vi "Emballage_BDD_option_Certificat.vi"(8 "Error in":errorcluster caption="Error in (no error)") -> (0 "Error out":errorcluster)   [LabVIEW 2020]
uses:
  Labview emballage/enum_ON_OFF_Lecteur.ctl
panel:
  in  "stop":bool
  in  "Bouton scanner":bool
  out "Code-barre":string
  # "Veuillez scanner le code-barre du produit!!"
  # "Attention: le produit scanné doit correspondre à la famille du produit de la commande en cours"
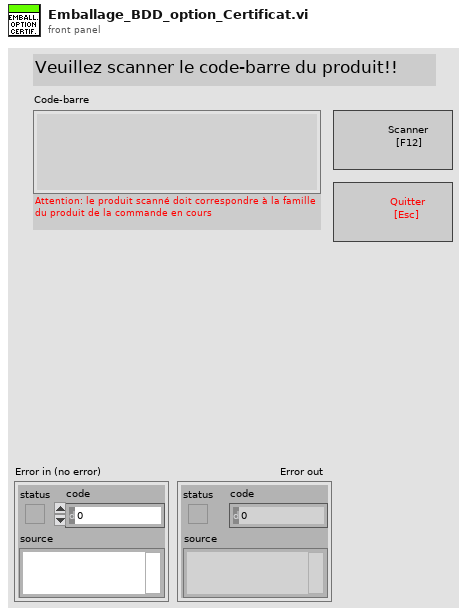
[diagram p1: front panel]
types:
  T1 = typedef "enum_ON_OFF_Lecteur.ctl" = enum16{"ON_COURT", "OFF", "ON", "OFF (open/Close)", "ON (open/close)"}
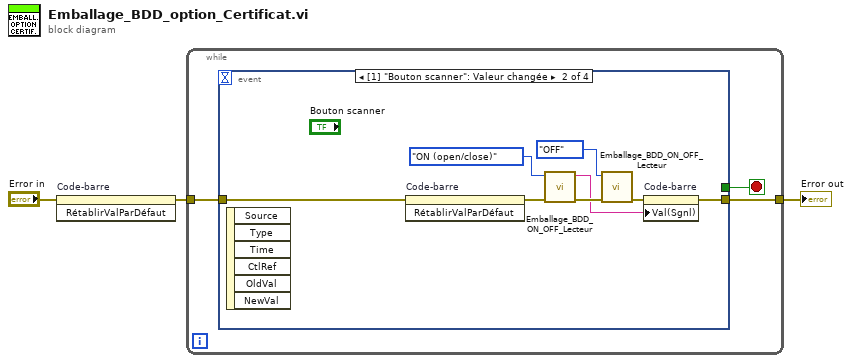
[diagram p0: block diagram]
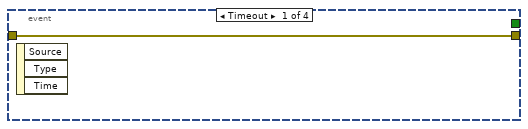
[diagram p2: hidden frame]
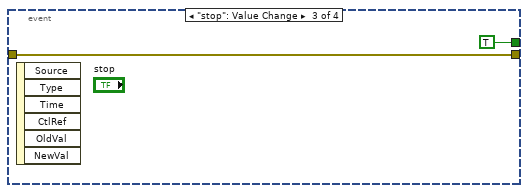
[diagram p3: hidden frame]
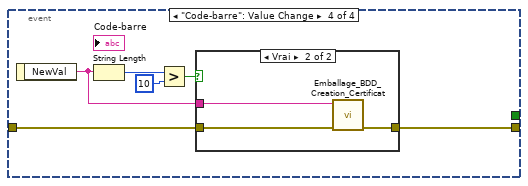
[diagram p4: hidden frame]
diagram:
  n1 = invoke on="Code-barre" class="Ch" method="RétablirValParDéfaut"(error in="Error in") -> (error out=w1:errorcluster)  [unwired: 2 in, 2 out]
  n2 = while {
    tunnel: w1 -> [w6]
    tunnel: [w5] -> w3
    stop <- w4 stop-if-true
    n3 = event shown="[1] \"Bouton scanner\": Valeur changée" {
      selector: _ -> [_ _ _ _]
      dyn-events: _ -> [_ _ _ _]
      timeout: _ -> [_ _ _ _]
      tunnel: w6 -> [w7 w12 w16 w23]
      tunnel: [w7 w9 w16 w22] -> w5
      tunnel: [_ _ TRUE _] -> w4
      event Timeout {
        n4 = event-data() -> ()  [unwired: 1 in, 3 out]
      }
      event "Bouton scanner": Value Change {
        n5 = event-data() -> ()  [unwired: 1 in, 6 out]
        n6 = invoke on="Code-barre" class="Ch" method="RétablirValParDéfaut"(error in=w12) -> (error out=w11:errorcluster)  [unwired: 2 in, 2 out]
        n7 = call "Emballage_BDD_ON_OFF_Lecteur.vi"("Error in"=w11, "ON/OFF lecteur"=enum_ON_OFF_Lecteur."ON (open/close)") -> ("Error out"=w14:errorcluster, "Etiquette scanné"=w8:string)  [unwired: 7 in, 1 out]
        n8 = call "Emballage_BDD_ON_OFF_Lecteur.vi"("Error in"=w14, "ON/OFF lecteur"=enum_ON_OFF_Lecteur."OFF") -> ("Error out"=w10:errorcluster)  [unwired: 7 in, 2 out]
        n9 = property on="Code-barre" class="Ch"(error in=w10, "Val(Sgnl)"=w8) -> (error out=w9:errorcluster)  [unwired: 1 in, 1 out]
      }
      event "stop": Value Change {
        n10 = event-data() -> ()  [unwired: 1 in, 6 out]
      }
      event "Code-barre": Value Change {
        n11 = event-data() -> ("NewVal"=w18:string)  [unwired: 1 in]
        n12 = String Length(string=w18) -> (length=w20:i32)
        n13 = Greater?(x=w20, y=10) -> (0:w19:bool)
        n14 = case shown="Vrai" w19 {
          tunnel: w18 -> [_ w27]
          tunnel: w23 -> [w24 w26]
          tunnel: [w24 w25] -> w22
          frame False {
          }
          frame True {
            n15 = call "Emballage_BDD_Creation_Certificat.vi"("Error in"=w26, "CODE BARRE du produit correspondant au certificat"=w27) -> ("Error out"=w25:errorcluster)  [unwired: 9 in]
          }
        }
      }
    }
  }
  "Error out" <- w3
